vi "GetType.vi"(8 "error in (no error)":errorcluster, 11 "Configure FM Source [FM] Msg in":refnum<class "Configure FM Source [FM] Msg.lvclass">) -> (0 "error out":errorcluster, 2 "Data Sample":variant, 3 "Configure FM Source [FM] Msg out":refnum<class "Configure FM Source [FM] Msg.lvclass">)   [LabVIEW 2014, in "CS++Fgen.lvlib" / "Configure FM Source [FM] Msg.lvclass"]
doc: "This VI delivers a sample of the data type format the message expects."
uses:
  Configure FM Source [FM] Msg.lvclass
  Configure FM Source [FM] Msg.lvclass/Configure FM Source [FM] Msg.ctl
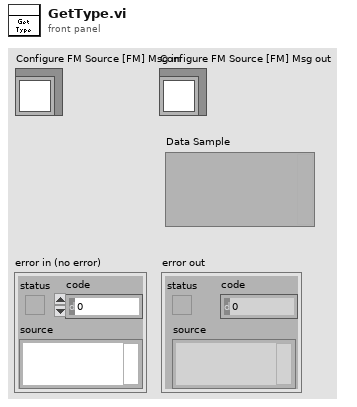
[diagram p1: front panel]
types:
  T1 = cluster{"Channel Name (\"\")":string, "source (Internal)":i32}
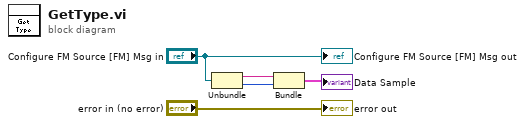
[diagram p0: block diagram]
diagram:
  n1 = Unbundle("Configure FM Source [FM] Msg in") -> (w3:string, w2:i32)
  n2 = Bundle("Channel Name (\"\")"=w3, "source (Internal)"=w2) -> (→"Data Sample":T1)  [unwired: 1 in]
  "error out" <- "error in (no error)"
  "Configure FM Source [FM] Msg out" <- "Configure FM Source [FM] Msg in"
